vi "Kill Actor.vi"(8 "error in (no error)":errorcluster) -> (0 "error out":errorcluster caption="sortie d'erreur")   [LabVIEW 2020, in "Library Core.lvlib" / "Sequencer (Default).lvclass"]
uses:
  Sequencer (Default).lvclass
  Actor Test (Default)/Actor Test (Default).lvclass
  Sequencer (Default).lvclass/Sequencer (Default).ctl
  Commun VI/Library Commun.lvlib
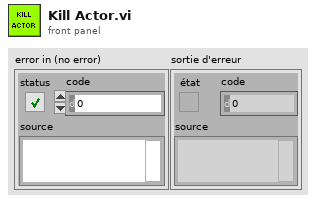
[diagram p1: front panel]
types:
  T1 = enum16{"Get Actor Class", "Set Actor object", "Get Actor object", "List Actor", "Init"}
  T2 = cluster{"Name":string, "Actor Test":refnum<class "Actor Test (Default).lvclass">}[]
  T3 = enum32{"Bad", "Idle", "Run top level", "Running"}
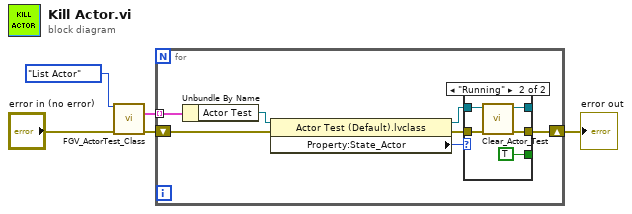
[diagram p0: block diagram]
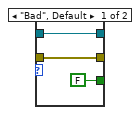
[diagram p2: hidden frame]
diagram:
  n1 = call "FGV_ActorTest_Class.vi"("Action"=T1."List Actor", "error in (no error)"="error in (no error)") -> ("List Test"=w5:T2, "error out"=w4:errorcluster)  [unwired: 10 in, 2 out]
  n2 = for {
    tunnel: w5 -> [w12] mode=indexing
    shift-right: [w6] -> w1
    shift-left: w4 -> [w10]
    n3 = Unbundle By Name(w12) -> ("Actor Test"=w11:refnum<class "Actor Test (Default).lvclass">)
    n4 = property class="Actor Test (Default).lvclass"(reference=w11, error in=w10) -> (reference out=w7:refnum<class "Actor Test (Default).lvclass">, error out=w9:errorcluster, "Property:State_Actor"=w8:T3)
    n5 = case shown="\"Running\"" w8 {
      tunnel: w7 -> [w15 w16]
      tunnel: w9 -> [w14 w19]
      tunnel: [w15 w17] -> _
      tunnel: [w14 w18] -> w6
      tunnel: [FALSE TRUE] -> _
      frame "Bad", Default {
      }
      frame "Running" {
        n6 = call-dynamic "Clear_Actor_Test.vi"("error in (no error)"=w19, "Test (Default) en entrée"=w16) -> ("error out"=w18:errorcluster, "Test (Default) en sortie"=w17:refnum<class "Actor Test (Default).lvclass">)  [unwired: 8 in]
      }
    }
  }
  "error out" <- w1
